vi "Write1ByteReg.vi"(7 "MxID":u8=254 format="%x", 8 "error in":errorcluster, 9 "Param":u8=2, 11 "RegAddr":u8=6 format="%x") -> (0 "error out":errorcluster, 3 "Data":u8[](array[numeric]) format="%x")   [LabVIEW 2014]
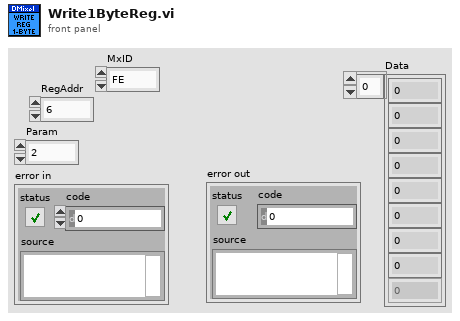
[diagram p1: front panel]
types:
  T1 = cluster{"MxID":u8, u8, u8, "RegAddr":u8, "Param":u8}
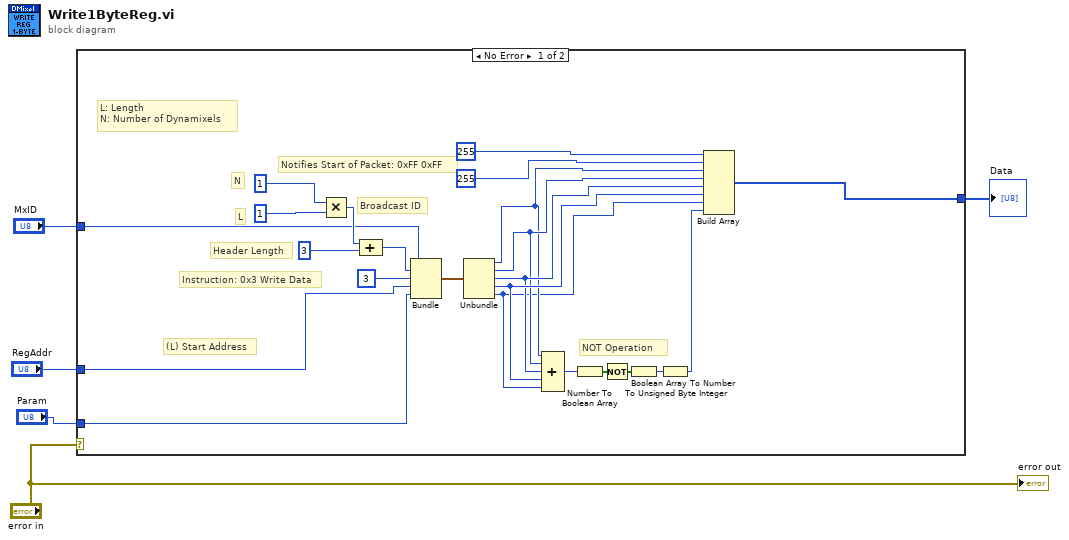
[diagram p0: block diagram]
diagram:
  n1 = case shown="No Error" "error in" {
    tunnel: "RegAddr" -> [w9 _]
    tunnel: [w15 _] -> w3
    tunnel: "MxID" -> [w10 _]
    tunnel: "Param" -> [w6 _]
    frame No Error {
      # "L"
      # "NOT Operation"
      # "L: Length \nN: Number of Dynamixels"
      # "Header Length"
      # "N"
      # "(L) Start Address"
      # "Instruction: 0x3 Write Data"
      # "Broadcast ID"
      # "Notifies Start of Packet: 0xFF 0xFF"
      n2 = Multiply(x=u8 1 ("N"), y=u8 1) -> (x*y=w28:u8)
      n3 = Compound Arithmetic op=unknown(w28, u8 3 ("value")) -> (w27:u8)
      n4 = Bundle("MxID"=w10, w27, u8 3, "RegAddr"=w9, "Param"=w6) -> (w23:T1)  [unwired: 1 in]
      n5 = Unbundle(w23) -> ("MxID"=w11:u8, w12:u8, w13:u8, "RegAddr"=w14:u8, "Param"=w8:u8)
      n6 = Compound Arithmetic op=ADD(w11, w12, w13, w14, w8) -> (w19:u8)
      n7 = Number To Boolean Array(number=w19) -> (Boolean array=w20:bool[])
      n8 = Not(x=w20) -> (.not. x?=w21:bool[])
      n9 = Boolean Array To Number(Boolean array=w21) -> (number=w22:u8)
      n10 = To Unsigned Byte Integer(number=w22) -> (unsigned 8bit integer=w7:u8)
      n11 = Build Array(u8 255, u8 255, w11, w12, w13, w14, w8, w7) -> (w15:u8[])
    }
    frame Error {
    }
  }
  "Data" <- w3
  "error out" <- "error in"
